vi "main(Test DQMH modules).vi"() -> ()   [LabVIEW 2018, in "Application.lvlib"] (continued)
              n429 = property class="ColBox"(reference=w1006, "Value"=u32 10000536 ("DRV 1")) -> ()  [unwired: 1 in, 2 out]
            }
            n430 = Build Array("Test Channel 2", "MEAS.AllRelaysOFF") -> (w1001:string[])
            n431 = for {
              tunnel: [w1010] -> w1002 mode=indexing
              tunnel: w1001 -> [w1009] mode=indexing
              tunnel: w1000 -> [w1008]
              n432 = call "App enquece.vi"("command"=w1009, "queue in"=w1008) -> ("error out"=w1010:errorcluster)  [unwired: 8 in, 1 out]
            }
            n433 = Merge Errors(w1004, w1002) -> (w1003:errorcluster)
          }
          event "Test Channel 3": Value Change {
            n434 = event-data() -> ()  [unwired: 1 in, 1 out]
            n435 = Array Subset(array=w1015, index=12, length=6) -> (w1016:refnum<vi>[])
            n436 = for {
              tunnel: w1016 -> [w1027] mode=indexing
              n437 = property class="ColBox"(reference=w1027, "Value"=u32 10000536 ("DRV 1")) -> ()  [unwired: 1 in, 2 out]
            }
            n438 = Build Array("Test Channel 3", "MEAS.AllRelaysOFF") -> (w1022:string[])
            n439 = for {
              tunnel: [w1031] -> w1023 mode=indexing
              tunnel: w1022 -> [w1030] mode=indexing
              tunnel: w1021 -> [w1029]
              n440 = call "App enquece.vi"("command"=w1030, "queue in"=w1029) -> ("error out"=w1031:errorcluster)  [unwired: 8 in, 1 out]
            }
            n441 = Merge Errors(w1025, w1023) -> (w1024:errorcluster)
          }
          event "Test Channel 4": Value Change {
            n442 = event-data() -> ()  [unwired: 1 in, 1 out]
            n443 = Array Subset(array=w1036, index=18, length=6) -> (w1037:refnum<vi>[])
            n444 = for {
              tunnel: w1037 -> [w1048] mode=indexing
              n445 = property class="ColBox"(reference=w1048, "Value"=u32 10000536 ("DRV 1")) -> ()  [unwired: 1 in, 2 out]
            }
            n446 = Build Array("Test Channel 4", "MEAS.AllRelaysOFF") -> (w1043:string[])
            n447 = for {
              tunnel: [w1052] -> w1044 mode=indexing
              tunnel: w1043 -> [w1051] mode=indexing
              tunnel: w1042 -> [w1050]
              n448 = call "App enquece.vi"("command"=w1051, "queue in"=w1050) -> ("error out"=w1052:errorcluster)  [unwired: 8 in, 1 out]
            }
            n449 = Merge Errors(w1046, w1044) -> (w1045:errorcluster)
          }
          event "Test Channel 5": Value Change {
            n450 = event-data() -> ()  [unwired: 1 in, 1 out]
            n451 = Array Subset(array=w1057, index=24, length=6) -> (w1058:refnum<vi>[])
            n452 = for {
              tunnel: w1058 -> [w1069] mode=indexing
              n453 = property class="ColBox"(reference=w1069, "Value"=u32 10000536 ("DRV 1")) -> ()  [unwired: 1 in, 2 out]
            }
            n454 = Build Array("Test Channel 5", "MEAS.AllRelaysOFF") -> (w1064:string[])
            n455 = for {
              tunnel: [w1073] -> w1065 mode=indexing
              tunnel: w1064 -> [w1072] mode=indexing
              tunnel: w1063 -> [w1071]
              n456 = call "App enquece.vi"("command"=w1072, "queue in"=w1071) -> ("error out"=w1073:errorcluster)  [unwired: 8 in, 1 out]
            }
            n457 = Merge Errors(w1067, w1065) -> (w1066:errorcluster)
          }
          event "Test Channel 6": Value Change {
            n458 = event-data() -> ()  [unwired: 1 in, 1 out]
            n459 = Array Subset(array=w1078, index=30, length=6) -> (w1079:refnum<vi>[])
            n460 = for {
              tunnel: w1079 -> [w1090] mode=indexing
              n461 = property class="ColBox"(reference=w1090, "Value"=u32 10000536 ("DRV 1")) -> ()  [unwired: 1 in, 2 out]
            }
            n462 = Build Array("Test Channel 6", "MEAS.AllRelaysOFF") -> (w1085:string[])
            n463 = for {
              tunnel: [w1094] -> w1086 mode=indexing
              tunnel: w1085 -> [w1093] mode=indexing
              tunnel: w1084 -> [w1092]
              n464 = call "App enquece.vi"("command"=w1093, "queue in"=w1092) -> ("error out"=w1094:errorcluster)  [unwired: 8 in, 1 out]
            }
            n465 = Merge Errors(w1088, w1086) -> (w1087:errorcluster)
          }
          event "Test Channel 7": Value Change {
            n466 = event-data() -> ()  [unwired: 1 in, 1 out]
            n467 = Array Subset(array=w1099, index=36, length=6) -> (w1100:refnum<vi>[])
            n468 = for {
              tunnel: w1100 -> [w1111] mode=indexing
              n469 = property class="ColBox"(reference=w1111, "Value"=u32 10000536 ("DRV 1")) -> ()  [unwired: 1 in, 2 out]
            }
            n470 = Build Array("Test Channel 7", "MEAS.AllRelaysOFF") -> (w1107:string[])
            n471 = for {
              tunnel: [w1115] -> w1103 mode=indexing
              tunnel: w1107 -> [w1114] mode=indexing
              tunnel: w1106 -> [w1113]
              n472 = call "App enquece.vi"("command"=w1114, "queue in"=w1113) -> ("error out"=w1115:errorcluster)  [unwired: 8 in, 1 out]
            }
            n473 = Merge Errors(w1109, w1103) -> (w1108:errorcluster)
          }
          event "Test Channel 8": Value Change {
            n474 = event-data() -> ()  [unwired: 1 in, 1 out]
            n475 = Array Subset(array=w1120, index=42, length=6) -> (w1121:refnum<vi>[])
            n476 = for {
              tunnel: w1121 -> [w1132] mode=indexing
              n477 = property class="ColBox"(reference=w1132, "Value"=u32 10000536 ("DRV 1")) -> ()  [unwired: 1 in, 2 out]
            }
            n478 = Build Array("Test Channel 8", "MEAS.AllRelaysOFF") -> (w1127:string[])
            n479 = for {
              tunnel: [w1136] -> w1128 mode=indexing
              tunnel: w1127 -> [w1135] mode=indexing
              tunnel: w1126 -> [w1134]
              n480 = call "App enquece.vi"("command"=w1135, "queue in"=w1134) -> ("error out"=w1136:errorcluster)  [unwired: 8 in, 1 out]
            }
            n481 = Merge Errors(w1130, w1128) -> (w1129:errorcluster)
          }
          event "Test Channel 9": Value Change {
            n482 = event-data() -> ()  [unwired: 1 in, 1 out]
            n483 = Array Subset(array=w1141, index=48, length=6) -> (w1142:refnum<vi>[])
            n484 = for {
              tunnel: w1142 -> [w1153] mode=indexing
              n485 = property class="ColBox"(reference=w1153, "Value"=u32 10000536 ("DRV 1")) -> ()  [unwired: 1 in, 2 out]
            }
            n486 = Build Array("Test Channel 9", "MEAS.AllRelaysOFF") -> (w1148:string[])
            n487 = for {
              tunnel: [w1157] -> w1149 mode=indexing
              tunnel: w1148 -> [w1156] mode=indexing
              tunnel: w1147 -> [w1155]
              n488 = call "App enquece.vi"("command"=w1156, "queue in"=w1155) -> ("error out"=w1157:errorcluster)  [unwired: 8 in, 1 out]
            }
            n489 = Merge Errors(w1151, w1149) -> (w1150:errorcluster)
          }
          event "Test Channel 10": Value Change {
            n490 = event-data() -> ()  [unwired: 1 in, 1 out]
            n491 = Array Subset(array=w1162, index=54, length=6) -> (w1163:refnum<vi>[])
            n492 = for {
              tunnel: w1163 -> [w1174] mode=indexing
              n493 = property class="ColBox"(reference=w1174, "Value"=u32 10000536 ("DRV 1")) -> ()  [unwired: 1 in, 2 out]
            }
            n494 = Build Array("Test Channel 10", "MEAS.AllRelaysOFF") -> (w1169:string[])
            n495 = for {
              tunnel: [w1178] -> w1170 mode=indexing
              tunnel: w1169 -> [w1177] mode=indexing
              tunnel: w1168 -> [w1176]
              n496 = call "App enquece.vi"("command"=w1177, "queue in"=w1176) -> ("error out"=w1178:errorcluster)  [unwired: 8 in, 1 out]
            }
            n497 = Merge Errors(w1172, w1170) -> (w1171:errorcluster)
          }
          event User Event {
            n498 = event-data() -> ("Init?"=w1182:bool)  [unwired: 1 in]
            "DC Measure Module" <- w1182
            "Inst. 1" <- w1182
            n499 = disable-structure shown="LOGGING==TRUE" {
              disable-tunnel: w1185 -> [w1192 _]
              frame condition #0 (active) {
                n500 = Empty String/Path?(string/path=w1192) -> (empty?=w1199:bool)
                n501 = Select(t="Quece timeout", s=w1199, f=w1192) -> (s? t:f=w1197:string)
                n502 = Format Into String(format string=":%s", initial string=w1197, "DMM  Did  it") -> (resulting string=w1194:string)  [unwired: 1 in, 1 out]
                n503 = call "string log (SubVI).vi"("Enum"=enum16{"Init", "Log", "Read"}."Log", "state Name"=w1194) -> ()  [unwired: 8 in, 2 out]
              }
              frame condition #1 {
              }
            }
            n504 = call "FGV Init phase.vi"("Boolean"=w1182) -> ("Init Completed?"=w1181:bool)  [unwired: 9 in, 1 out]
            n505 = case shown="True" w1181 {
              tunnel: w1180 -> [_ w1191]
              frame False {
              }
              frame True {
                n506 = call "App enquece.vi"("command"="INIT.Read DRV code", "queue in"=w1191) -> ()  [unwired: 8 in, 2 out]
              }
            }
            n507 = disable-structure shown="DEBUGGING==TRUE" {
              disable-tunnel: [w1200 w1202] -> w1187
              disable-tunnel: w1186 -> [w1200 w1203]
              frame condition #0 (active) {
              }
              frame condition #1 {
                n508 = call "Show Panel.vi"() -> ("error out"=w1201:errorcluster)  [unwired: 11 in]
                n509 = Merge Errors(w1203, w1201) -> (w1202:errorcluster)
              }
            }
          }
          event User Event {
            n510 = event-data() -> ("Init?"=w1207:bool)  [unwired: 1 in]
            "AC switches Module" <- w1207
            "Inst. 2" <- w1207
            n511 = disable-structure shown="LOGGING==TRUE" {
              disable-tunnel: w1212 -> [w1221 _]
              frame condition #0 (active) {
                n512 = Empty String/Path?(string/path=w1221) -> (empty?=w1228:bool)
                n513 = Select(t="Quece timeout", s=w1228, f=w1221) -> (s? t:f=w1226:string)
                n514 = Format Into String(format string=":%s", initial string=w1226, "MB01  Did  it") -> (resulting string=w1223:string)  [unwired: 1 in, 1 out]
                n515 = call "string log (SubVI).vi"("Enum"=enum16{"Init", "Log", "Read"}."Log", "state Name"=w1223) -> ()  [unwired: 8 in, 2 out]
              }
              frame condition #1 {
              }
            }
            n516 = call "FGV Init phase.vi"("Boolean"=w1207) -> ("Init Completed?"=w1206:bool)  [unwired: 9 in, 1 out]
            n517 = disable-structure shown="DEBUGGING==TRUE" {
              disable-tunnel: [w1217 w1220] -> w1211
              disable-tunnel: w1210 -> [w1217 w1219]
              frame condition #0 (active) {
              }
              frame condition #1 {
                n518 = call "Show Panel.vi"() -> ("error out"=w1218:errorcluster)  [unwired: 11 in]
                n519 = Merge Errors(w1219, w1218) -> (w1220:errorcluster)
              }
            }
            n520 = case shown="True" w1206 {
              tunnel: w1205 -> [_ w1215]
              frame False {
              }
              frame True {
                n521 = call "App enquece.vi"("command"="INIT.Read DRV code", "queue in"=w1215) -> ()  [unwired: 8 in, 2 out]
              }
            }
          }
          event User Event {
            n522 = event-data() -> ("Init?"=w1232:bool)  [unwired: 1 in]
            "DC Switches Module" <- w1232
            "Inst. 3" <- w1232
            n523 = disable-structure shown="LOGGING==TRUE" {
              disable-tunnel: w1235 -> [w1242 _]
              frame condition #0 (active) {
                n524 = Empty String/Path?(string/path=w1242) -> (empty?=w1249:bool)
                n525 = Select(t="Quece timeout", s=w1249, f=w1242) -> (s? t:f=w1247:string)
                n526 = Format Into String(format string=":%s", initial string=w1247, "M054  Did  it") -> (resulting string=w1244:string)  [unwired: 1 in, 1 out]
                n527 = call "string log (SubVI).vi"("Enum"=enum16{"Init", "Log", "Read"}."Log", "state Name"=w1244) -> ()  [unwired: 8 in, 2 out]
              }
              frame condition #1 {
              }
            }
            n528 = call "FGV Init phase.vi"("Boolean"=w1232) -> ("Init Completed?"=w1231:bool)  [unwired: 9 in, 1 out]
            n529 = case shown="True" w1231 {
              tunnel: w1230 -> [_ w1240]
              frame False {
              }
              frame True {
                n530 = call "App enquece.vi"("command"="INIT.Read DRV code", "queue in"=w1240) -> ()  [unwired: 8 in, 2 out]
              }
            }
            n531 = disable-structure shown="DEBUGGING==TRUE" {
              disable-tunnel: w1237 -> [w1250 w1252 w1255]
              disable-tunnel: [w1251 w1252 w1253] -> w1236
              frame condition #0 (active) {
                n532 = Merge Errors(w1250) -> (w1251:errorcluster)
              }
              frame condition #1 {
              }
              frame condition #2 {
                n533 = call "Show Panel.vi"() -> ("error out"=w1254:errorcluster)  [unwired: 11 in]
                n534 = Merge Errors(w1255, w1254) -> (w1253:errorcluster)
              }
            }
          }
        }
      }
      frame "Apps.AutoMode" {
        # "Check Jig trigger every 100ms"
        n535 = disable-structure shown="Enabled" {
          frame Disabled {
            n536 = local write "Auto/Man"(TRUE) -> ()
          }
          frame Enabled {
          }
        }
      }
      frame "Apps.WaitingForTrigger" {
        n537 = call "App enquece.vi"("command"="MEAS.Read TRIGGER", "queue in"=w1270) -> ("error out"=w1268:errorcluster)  [unwired: 8 in, 1 out]
        n538 = Merge Errors(w1266, w1268) -> (w1267:errorcluster)
      }
      frame "Apps.UpdateStatus" {
        n539 = disable-structure shown="LOGGING==TRUE" {
          disable-tunnel: w1278 -> [w1291 _]
          frame condition #0 (active) {
            n540 = Empty String/Path?(string/path=w1291) -> (empty?=w1294:bool)
            n541 = Select(t="Quece timeout", s=w1294, f=w1291) -> (s? t:f=w1290:string)
            n542 = call "string log (SubVI).vi"("Enum"=enum16{"Init", "Log", "Read"}."Log", "state Name"=w1290) -> ()  [unwired: 8 in, 2 out]
          }
          frame condition #1 {
          }
        }
        n543 = call "App enquece.vi"("command"="Apps.WaitForEvent", "queue in"=w1286) -> ("error out"=w1283:errorcluster)  [unwired: 8 in, 1 out]
        n544 = Merge Errors(w1279, w1283) -> (w1280:errorcluster)
      }
      frame "Apps.UI Update" {
        # "Update UI  6LED (channel)"
        n545 = disable-structure shown="LOGGING==TRUE" {
          disable-tunnel: w1298 -> [w1418 _]
          frame condition #0 (active) {
            n546 = Empty String/Path?(string/path=w1418) -> (empty?=w1421:bool)
            n547 = Select(t="Quece timeout", s=w1421, f=w1418) -> (s? t:f=w1417:string)
            n548 = call "string log (SubVI).vi"("Enum"=enum16{"Init", "Log", "Read"}."Log", "state Name"=w1417) -> ()  [unwired: 8 in, 2 out]
          }
          frame condition #1 {
          }
        }
        n549 = Variant To Data(type="", Variant=w1296) -> (data=w1295:string)  [unwired: 1 in, 1 out]
        n550 = case shown="\"A\"" w1295 {
          tunnel: [w1319 w1327 w1345 w1363 w1381 w1399] -> w1304
          tunnel: w1302 -> [w1317 w1328 w1346 w1364 w1382 w1400]
          tunnel: w1301 -> [w1314 w1329 w1347 w1365 w1383 w1401]
          frame "", Default {
            w1311 = 6 ("length")
            n551 = call "FGV Driver Data.vi"("DUT channel (1-11)"=w1314, "FGV enum(Read)"=FGV_DRV_data."Process" ("FGV DRV data enum")) -> ("60 DRV data"=w1312:T17[])  [unwired: 6 in, 3 out]
            n552 = Decrement(x=w1314) -> (x-1=w1315:i32)
            n553 = Multiply(x=w1315, y=w1311) -> (x*y=w1313:i32)
            n554 = Array Subset(array=w1312, index=w1313, length=w1311) -> (w1310:T17[])
            n555 = Array Subset(array=w1317, index=w1313, length=w1311) -> (w1316:refnum<vi>[])
            n556 = for {
              tunnel: w1316 -> [w1322] mode=indexing
              tunnel: w1310 -> [w1321] mode=indexing
              tunnel: [w1320] -> w1319 mode=indexing
              n557 = Unbundle By Name(w1321) -> ("DRV Fail/Pass (T)"=w1325:bool)
              n558 = Select(t=u32 16711686 ("DRV 1"), s=w1325, f=u32 65309 ("DRV 1")) -> (s? t:f=w1326:u32)
              n559 = property class="ColBox"(reference=w1322, "Value"=w1326) -> (error out=w1320:errorcluster)  [unwired: 1 in, 1 out]
            }
          }
          frame "A" {
            w1330 = 1
            n560 = call "FGV Driver Data.vi"("DUT channel (1-11)"=w1329, "FGV enum(Read)"=FGV_DRV_data."Process" ("FGV DRV data enum")) -> ("60 DRV data"=w1333:T17[])  [unwired: 6 in, 3 out]
            n561 = Decrement(x=w1329) -> (x-1=w1335:i32)
            n562 = Multiply(x=w1335, y=6 ("length")) -> (x*y=w1334:i32)
            n563 = Array Subset(array=w1333, index=w1334, length=w1330) -> (w1331:T17[])
            n564 = Array Subset(array=w1328, index=w1334, length=w1330) -> (w1336:refnum<vi>[])
            n565 = for {
              tunnel: w1336 -> [w1340] mode=indexing
              tunnel: w1331 -> [w1339] mode=indexing
              tunnel: [w1338] -> w1327 mode=indexing
              n566 = Unbundle By Name(w1339) -> ("DRV Fail/Pass (T)"=w1343:bool)
              n567 = Select(t=u32 16711686 ("DRV 1"), s=w1343, f=u32 65309 ("DRV 1")) -> (s? t:f=w1344:u32)
              n568 = property class="ColBox"(reference=w1340, "Value"=w1344) -> (error out=w1338:errorcluster)  [unwired: 1 in, 1 out]
            }
          }
          frame "B" {
            w1348 = 2
            n569 = call "FGV Driver Data.vi"("DUT channel (1-11)"=w1347, "FGV enum(Read)"=FGV_DRV_data."Process" ("FGV DRV data enum")) -> ("60 DRV data"=w1351:T17[])  [unwired: 6 in, 3 out]
            n570 = Decrement(x=w1347) -> (x-1=w1353:i32)
            n571 = Multiply(x=w1353, y=6 ("length")) -> (x*y=w1352:i32)
            n572 = Array Subset(array=w1351, index=w1352, length=w1348) -> (w1349:T17[])
            n573 = Array Subset(array=w1346, index=w1352, length=w1348) -> (w1354:refnum<vi>[])
            n574 = for {
              tunnel: w1354 -> [w1358] mode=indexing
              tunnel: w1349 -> [w1357] mode=indexing
              tunnel: [w1356] -> w1345 mode=indexing
              n575 = Unbundle By Name(w1357) -> ("DRV Fail/Pass (T)"=w1361:bool)
              n576 = Select(t=u32 16711686 ("DRV 1"), s=w1361, f=u32 65309 ("DRV 1")) -> (s? t:f=w1362:u32)
              n577 = property class="ColBox"(reference=w1358, "Value"=w1362) -> (error out=w1356:errorcluster)  [unwired: 1 in, 1 out]
            }
          }
          frame "C" {
            w1366 = 3
            n578 = call "FGV Driver Data.vi"("DUT channel (1-11)"=w1365, "FGV enum(Read)"=FGV_DRV_data."Process" ("FGV DRV data enum")) -> ("60 DRV data"=w1369:T17[])  [unwired: 6 in, 3 out]
            n579 = Decrement(x=w1365) -> (x-1=w1371:i32)
            n580 = Multiply(x=w1371, y=6 ("length")) -> (x*y=w1370:i32)
            n581 = Array Subset(array=w1369, index=w1370, length=w1366) -> (w1367:T17[])
            n582 = Array Subset(array=w1364, index=w1370, length=w1366) -> (w1372:refnum<vi>[])
            n583 = for {
              tunnel: w1372 -> [w1376] mode=indexing
              tunnel: w1367 -> [w1375] mode=indexing
              tunnel: [w1374] -> w1363 mode=indexing
              n584 = Unbundle By Name(w1375) -> ("DRV Fail/Pass (T)"=w1379:bool)
              n585 = Select(t=u32 16711686 ("DRV 1"), s=w1379, f=u32 65309 ("DRV 1")) -> (s? t:f=w1380:u32)
              n586 = property class="ColBox"(reference=w1376, "Value"=w1380) -> (error out=w1374:errorcluster)  [unwired: 1 in, 1 out]
            }
          }
          frame "D" {
            w1384 = 4
            n587 = call "FGV Driver Data.vi"("DUT channel (1-11)"=w1383, "FGV enum(Read)"=FGV_DRV_data."Process" ("FGV DRV data enum")) -> ("60 DRV data"=w1387:T17[])  [unwired: 6 in, 3 out]
            n588 = Decrement(x=w1383) -> (x-1=w1389:i32)
            n589 = Multiply(x=w1389, y=6 ("length")) -> (x*y=w1388:i32)
            n590 = Array Subset(array=w1387, index=w1388, length=w1384) -> (w1385:T17[])
            n591 = Array Subset(array=w1382, index=w1388, length=w1384) -> (w1390:refnum<vi>[])
            n592 = for {
              tunnel: w1390 -> [w1394] mode=indexing
              tunnel: w1385 -> [w1393] mode=indexing
              tunnel: [w1392] -> w1381 mode=indexing
              n593 = Unbundle By Name(w1393) -> ("DRV Fail/Pass (T)"=w1397:bool)
              n594 = Select(t=u32 16711686 ("DRV 1"), s=w1397, f=u32 65309 ("DRV 1")) -> (s? t:f=w1398:u32)
              n595 = property class="ColBox"(reference=w1394, "Value"=w1398) -> (error out=w1392:errorcluster)  [unwired: 1 in, 1 out]
            }
          }
          frame "E" {
            w1402 = 5
            n596 = call "FGV Driver Data.vi"("DUT channel (1-11)"=w1401, "FGV enum(Read)"=FGV_DRV_data."Process" ("FGV DRV data enum")) -> ("60 DRV data"=w1405:T17[])  [unwired: 6 in, 3 out]
            n597 = Decrement(x=w1401) -> (x-1=w1407:i32)
            n598 = Multiply(x=w1407, y=6 ("length")) -> (x*y=w1406:i32)
            n599 = Array Subset(array=w1405, index=w1406, length=w1402) -> (w1403:T17[])
            n600 = Array Subset(array=w1400, index=w1406, length=w1402) -> (w1408:refnum<vi>[])
            n601 = for {
              tunnel: w1408 -> [w1412] mode=indexing
              tunnel: w1403 -> [w1411] mode=indexing
              tunnel: [w1410] -> w1399 mode=indexing
              n602 = Unbundle By Name(w1411) -> ("DRV Fail/Pass (T)"=w1415:bool)
              n603 = Select(t=u32 16711686 ("DRV 1"), s=w1415, f=u32 65309 ("DRV 1")) -> (s? t:f=w1416:u32)
              n604 = property class="ColBox"(reference=w1412, "Value"=w1416) -> (error out=w1410:errorcluster)  [unwired: 1 in, 1 out]
            }
          }
        }
        n605 = Merge Errors(w1305, w1304) -> (w1306:errorcluster)
      }
      frame "Apps.UI Update 1" {
        # "For Update UI 1 LED"
        n606 = disable-structure shown="LOGGING==TRUE" {
          disable-tunnel: w1436 -> [w1444 _]
          frame condition #0 (active) {
            n607 = Empty String/Path?(string/path=w1444) -> (empty?=w1447:bool)
            n608 = Select(t="Quece timeout", s=w1447, f=w1444) -> (s? t:f=w1443:string)
            n609 = call "string log (SubVI).vi"("Enum"=enum16{"Init", "Log", "Read"}."Log", "state Name"=w1443) -> ()  [unwired: 8 in, 2 out]
          }
          frame condition #1 {
          }
        }
        n610 = call "FGV Driver Data.vi"("DUT channel (1-11)"=w1434, "FGV enum(Read)"=FGV_DRV_data."Process" ("FGV DRV data enum")) -> ("60 DRV data"=w1427:T17[])  [unwired: 6 in, 3 out]
        n611 = Decrement(x=w1422) -> (x-1=w1423:i32)
        n612 = Index Array(array=w1428, index=w1423) -> (element=w1425:refnum<vi>)
        n613 = Index Array(array=w1427, index=w1423) -> (element=w1426:T17)
        n614 = Unbundle By Name(w1426) -> ("DRV Fail/Pass (T)"=w1424:bool)
        n615 = Select(t=u32 16711686 ("DRV 1"), s=w1424, f=u32 65309 ("DRV 1")) -> (s? t:f=w1431:u32)
        n616 = property class="ColBox"(reference=w1425, "Value"=w1431) -> (error out=w1437:errorcluster)  [unwired: 1 in, 1 out]
        n617 = Merge Errors(w1438, w1437) -> (w1439:errorcluster)
      }
      frame "Apps.UI Update 2" {
        # "For Updat PCB OK/NG (1 LED)"
        n618 = local read "Auto/Man"() -> (w1455:bool)
        n619 = disable-structure shown="LOGGING==TRUE" {
          disable-tunnel: w1468 -> [w1510 _]
          frame condition #0 (active) {
            n620 = Empty String/Path?(string/path=w1510) -> (empty?=w1513:bool)
            n621 = Select(t="Quece timeout", s=w1513, f=w1510) -> (s? t:f=w1509:string)
            n622 = call "string log (SubVI).vi"("Enum"=enum16{"Init", "Log", "Read"}."Log", "state Name"=w1509) -> ()  [unwired: 8 in, 2 out]
          }
          frame condition #1 {
          }
        }
        n623 = case shown="True" w1455 {
          tunnel: w1460 -> [_ w1502]
          tunnel: [_ w1501] -> w1459
          frame False {
          }
          frame True {
            n624 = call "App enquece.vi"("command"="Apps.AutoMode", "queue in"=w1502) -> ("error out"=w1501:errorcluster)  [unwired: 8 in, 1 out]
          }
        }
        n625 = call "FGV Driver Data.vi"("error in (no error)"=w1459, "FGV enum(Read)"=FGV_DRV_data."Process" ("FGV DRV data enum")) -> ("error out"=w1467:errorcluster, "60 DRV data"=w1464:T17[])  [unwired: 6 in, 2 out]
        n626 = call "FGV DUT steps.vi"("Enum"=enum16{"write", "read"}."read") -> ("Steps OUT"=w1452:string[])  [unwired: 10 in]
        n627 = Index Array(array=w1452, index=1) -> (element=w1453:string)
        n628 = Decimal String To Number(string=w1453) -> (number=w1450:i32)  [unwired: 2 in, 1 out]
        n629 = call "find Index and length.vi"("number of DRV"=w1450) -> ("length"=w1448:i32, "index"=w1449:i32)  [unwired: 8 in, 1 out]
        n630 = disable-structure shown="Enabled" {
          disable-tunnel: w1464 -> [w1484 w1499]
          disable-tunnel: [w1482 w1498] -> w1457
          disable-tunnel: w1449 -> [_ w1497]
          disable-tunnel: w1448 -> [_ w1496]
          frame Disabled {
            n631 = local read "Enum"() -> (w1483:T1)
            n632 = case shown="\"00037845(M26)\"" w1483 {
              tunnel: w1484 -> [w1487 w1489 w1491 w1495]
              tunnel: [w1486 w1488 w1491 w1494] -> w1482
              frame "Fixxed", Default {
                n633 = Array Subset(array=w1487, length=41) -> (w1486:T17[])  [unwired: 1 in]
              }
              frame "Pinpoint_JIG" {
                n634 = Array Subset(array=w1489, index=42) -> (w1488:T17[])  [unwired: 1 in]
              }
              frame "All DRV" {
              }
              frame "00037845(M26)" {
                n635 = Array Subset(array=w1495, index=42, length=14) -> (w1494:T17[])
              }
            }
          }
          frame Enabled {
            n636 = Array Subset(array=w1499, index=w1497, length=w1496) -> (w1498:T17[])
          }
        }
        n637 = for {
          tunnel: w1457 -> [w1515] mode=indexing
          tunnel: [w1514] -> w1474 mode=indexing
          n638 = Unbundle By Name(w1515) -> ("DRV Fail/Pass (T)"=w1514:bool)
        }
        n639 = Or Array Elements(Boolean array=w1474) -> (logical OR=w1472:bool)
        n640 = control-ref of="DRV 61"() -> (w1473:refnum<vi>)
        n641 = Select(t=u32 16711680 ("DRV 1"), s=w1472, f=u32 6618880 ("DRV 1")) -> (s? t:f=w1469:u32)
        n642 = property class="ColBox"(reference=w1473, error in=w1467, "Value"=w1469) -> (error out=w1466:errorcluster)  [unwired: 1 out]
        n643 = case shown="False" "Log report" {
          tunnel: w1457 -> [_ w1504]
          tunnel: w1456 -> [_ w1505]
          frame False {
          }
          frame True {
            # "Log trigger"
            n644 = To Variant(anything=w1504) -> (Variant=w1503:variant)
            n645 = Enqueue Element(queue=w1505, element=w1503) -> ()  [unwired: 2 in, 3 out]
          }
        }
        n646 = Merge Errors(w1481, w1466) -> (w1461:errorcluster)
        n647 = disable-structure shown="NO_HARDWARE==TRUE" {
          disable-tunnel: [w1506 w1508] -> w1462
          disable-tunnel: w1461 -> [w1506 w1508]
          frame condition #0 (active) {
            n648 = Wait (ms)(milliseconds to wait=u32 2000) -> ()  [unwired: 1 out]
          }
          frame condition #1 {
          }
        }
      }
      frame "Apps.UI Update SC" {
        w1525 = "All Shorted Circuits"
        n649 = disable-structure shown="LOGGING==TRUE" {
          disable-tunnel: w1531 -> [w1576 _]
          frame condition #0 (active) {
            n650 = Empty String/Path?(string/path=w1576) -> (empty?=w1579:bool)
            n651 = Select(t="Quece timeout", s=w1579, f=w1576) -> (s? t:f=w1575:string)
            n652 = call "string log (SubVI).vi"("Enum"=enum16{"Init", "Log", "Read"}."Log", "state Name"=w1575) -> ()  [unwired: 8 in, 2 out]
          }
          frame condition #1 {
          }
        }
        n653 = call "FGV DUT steps.vi"("Enum"=enum16{"write", "read"}."read") -> ("Steps OUT"=w1517:string[])  [unwired: 10 in]
        n654 = Index Array(array=w1517, index=1) -> (element=w1519:string)
        n655 = call "FGV Driver Data.vi"("FGV enum(Read)"=FGV_DRV_data."Read" ("FGV DRV data enum")) -> ("60 DRV data"=w1522:T17[])  [unwired: 7 in, 3 out]
        n656 = Decimal String To Number(string=w1519) -> (number=w1518:i32)  [unwired: 2 in, 1 out]
        n657 = disable-structure shown="Enabled" {
          disable-tunnel: w1524 -> [w1544 w1568]
          disable-tunnel: [w1543 w1567] -> w1523
          disable-tunnel: w1522 -> [w1542 w1566]
          disable-tunnel: [w1541 w1563] -> w1521
          disable-tunnel: w1518 -> [_ w1569]
          frame Disabled {
            n658 = local read "Enum"() -> (w1540:T1)
            n659 = case shown="\"00037845(M26)\"" w1540 {
              tunnel: w1544 -> [w1549 w1554 w1556 w1561]
              tunnel: [w1548 w1550 w1556 w1559] -> w1543
              tunnel: w1542 -> [w1547 w1553 w1555 w1560]
              tunnel: [w1545 w1552 w1555 w1558] -> w1541
              frame "Fixxed", Default {
                w1546 = 42 ("length")
                n660 = Array Subset(array=w1547, length=w1546) -> (w1545:T17[])  [unwired: 1 in]
                n661 = Array Subset(array=w1549, length=w1546) -> (w1548:refnum<vi>[])  [unwired: 1 in]
              }
              frame "Pinpoint_JIG" {
                w1551 = 42 ("length")
                n662 = Array Subset(array=w1554, index=w1551) -> (w1550:refnum<vi>[])  [unwired: 1 in]
                n663 = Array Subset(array=w1553, index=w1551) -> (w1552:T17[])  [unwired: 1 in]
              }
              frame "All DRV" {
              }
              frame "00037845(M26)" {
                w1557 = 14 ("length")
                w1562 = 42 ("length")
                n664 = Array Subset(array=w1561, index=w1562, length=w1557) -> (w1559:refnum<vi>[])
                n665 = Array Subset(array=w1560, index=w1562, length=w1557) -> (w1558:T17[])
              }
            }
          }
          frame Enabled {
            n666 = call "find Index and length.vi"("number of DRV"=w1569) -> ("length"=w1564:i32, "index"=w1565:i32)  [unwired: 8 in, 1 out]
            n667 = Array Subset(array=w1568, index=w1565, length=w1564) -> (w1567:refnum<vi>[])
            n668 = Array Subset(array=w1566, index=w1565, length=w1564) -> (w1563:T17[])
          }
        }
        n669 = for {
          tunnel: w1521 -> [w1586] mode=indexing
          tunnel: w1523 -> [w1581] mode=indexing
          tunnel: [w1580] -> w1529 mode=indexing
          n670 = Unbundle By Name(w1586) -> ("Shorted Circuit"=w1582:bool)
          n671 = Select(t=u32 16711680 ("DRV 1"), s=w1582, f=u32 6618880 ("DRV 1")) -> (s? t:f=w1585:u32)
          n672 = property class="ColBox"(reference=w1581, "Value"=w1585) -> (error out=w1580:errorcluster)  [unwired: 1 in, 1 out]
        }
        n673 = Merge Errors(w1529) -> (w1528:errorcluster)
        n674 = flat-sequence {
          tunnel: w1528 -> [w1571]
          tunnel: [w1571] -> w1527
          tunnel: w1527 -> [w1573]
          tunnel: [w1574] -> w1526
          tunnel: w1524 -> [w1572]
          frame #0 {
            n675 = Wait (ms)(milliseconds to wait=u32 1500) -> ()  [unwired: 1 out]
          }
          frame #1 {
            n676 = call "reset DRV UI (SubVI).vi"("error in (no error)"=w1573, "Ref  in"=w1572) -> ("error out"=w1574:errorcluster)  [unwired: 8 in, 1 out]
          }
        }
        n677 = Merge Errors(w1539, w1526) -> (w1530:errorcluster)
        n678 = local write "Progress"(w1525) -> ()
      }
      frame "Timer Start" {
        n679 = flat-sequence {
          tunnel: [u32 0 ("time elased(ms)")] -> w1587
          frame #0 {
            n680 = call "FGV milisec (subVI).vi"() -> ()  [unwired: 11 in, 1 out]
          }
        }
        n681 = local write "time elased(ms)"(w1587) -> ()
      }
      frame "Timer Stop" {
        n682 = flat-sequence {
          tunnel: [w1608] -> w1597
          tunnel: w1598 -> [w1608]
          tunnel: [w1607] -> w1599
          frame #0 {
            n683 = call "FGV milisec (subVI).vi"() -> ("Elased Time (ms)"=w1607:u32)  [unwired: 11 in]
          }
        }
        "time elased(ms)" <- w1599
      }
      frame "WaitFor" {
        n684 = Variant To Data(type=u32 0, Variant=w1609) -> ()  [unwired: 1 in, 2 out]
        n685 = Wait (ms)(milliseconds to wait="milliseconds to wait") -> ()  [unwired: 1 out]
      }
      frame "Apps.Exit" {
        w1624 = TRUE
        n686 = disable-structure shown="LOGGING==TRUE" {
          disable-tunnel: w1621 -> [w1639 _]
          frame condition #0 (active) {
            n687 = Empty String/Path?(string/path=w1639) -> (empty?=w1642:bool)
            n688 = Select(t="Quece timeout", s=w1642, f=w1639) -> (s? t:f=w1638:string)
            n689 = call "string log (SubVI).vi"("Enum"=enum16{"Init", "Log", "Read"}."Log", "state Name"=w1638) -> ()  [unwired: 8 in, 2 out]
          }
          frame condition #1 {
          }
        }
        n690 = call "Application Name--constant.vi"() -> ("Application Name"=w1625:string)  [unwired: 11 in]
        n691 = call "Stop Module.vi"("Wait for Module to stop? (F)"=w1624, "Origin"=w1625, "Module ID"=-1) -> ("error out"=w1627:errorcluster)  [unwired: 8 in]
        n692 = call "Stop Module.vi"("Wait for Module to Stop? (F)"=w1624, "Origin"=w1625) -> ("error out"=w1633:errorcluster)  [unwired: 9 in]
        n693 = call "Stop Module.vi"("Wait for Module to Stop? (F)"=w1624, "Origin"=w1625) -> ("error out"=w1632:errorcluster)  [unwired: 9 in]
        n694 = call "Stop Module.vi"("Wait for Module to Stop? (F)"=w1624, "Origin"=w1625) -> ("error out"=w1631:errorcluster)  [unwired: 9 in]
        n695 = Merge Errors(w1629, w1633, w1632, w1631, w1627) -> (w1630:errorcluster)
      }
      frame "Apps.Error Handler" {
        w1651 = TRUE  # Priority Enquece
        n696 = disable-structure shown="LOGGING==TRUE" {
          disable-tunnel: w1644 -> [w1660 _]
          frame condition #0 (active) {
            n697 = Empty String/Path?(string/path=w1660) -> (empty?=w1663:bool)
            n698 = Select(t="Quece timeout", s=w1663, f=w1660) -> (s? t:f=w1659:string)
            n699 = call "string log (SubVI).vi"("Enum"=enum16{"Init", "Log", "Read"}."Log", "state Name"=w1659) -> ()  [unwired: 8 in, 2 out]
          }
          frame condition #1 {
          }
        }
        n700 = call <vilib>:"Simple Error Handler.vi"("error in (no error)"=w1658) -> ("error out"=w1653:errorcluster)  [unwired: 4 in, 4 out]
        n701 = flat-sequence {
          tunnel: w1653 -> [_]
          tunnel: [w1664] -> w1645
          frame #0 {
            n702 = xnode "Error Ring"() -> ("error out"=w1664:errorcluster)
          }
        }
        n703 = call "App enquece.vi"("Priority Enquece"=w1651, "command"="Apps.Exit", "queue in"=w1652) -> ("error out"=w1650:errorcluster)  [unwired: 7 in, 1 out]
        n704 = Merge Errors(w1645, w1650) -> (w1646:errorcluster)
      }
      frame "INIT.Init FGV" {
        n705 = call "FGV_HoldingRegs.vi"("FGV_enum"=FGV_enum."Init FGV") -> ("error out"=w1670:errorcluster)  [unwired: 8 in, 2 out]
        n706 = call "string log (SubVI).vi"("error in (no error)"=w1670, "Enum"=enum16{"Init", "Log", "Read"}."Init") -> ("error out"=w1671:errorcluster)  [unwired: 8 in, 1 out]
        n707 = call "FGV Driver Data.vi"("error in (no error)"=w1671, "FGV enum(Read)"=FGV_DRV_data."Init" ("FGV DRV data enum")) -> ("error out"=w1668:errorcluster)  [unwired: 6 in, 3 out]
        n708 = call "FGV Init phase.vi"("error in (no error)"=w1668, "FGV Enum"=enum16{"Init", "Check"}."Init") -> ("error out"=w1666:errorcluster)  [unwired: 8 in, 1 out]
        n709 = flat-sequence {
          tunnel: [w1684] -> w1667
          tunnel: w1666 -> [w1684]
          frame #0 {
            n710 = Initialize Array(FALSE, 6 ("dimension size"), 10 ("dimension size")) -> (w1688:bool[][])
            n711 = local write "EMIC connected"(bool[] [FALSE, FALSE, FALSE, FALSE, FALSE, FALSE] ("Array")) -> ()
            n712 = local write "Auto/Man"(FALSE) -> ()
            n713 = local write "Short DRV"(w1688) -> ()
          }
        }
        n714 = Merge Errors(w1683, w1667) -> (w1673:errorcluster)
      }
      frame "INIT.Read HW config" {
        n715 = disable-structure shown="LOGGING==TRUE" {
          disable-tunnel: w1703 -> [w1729 _]
          frame condition #0 (active) {
            n716 = Empty String/Path?(string/path=w1729) -> (empty?=w1732:bool)
            n717 = Select(t="Quece timeout", s=w1732, f=w1729) -> (s? t:f=w1728:string)
            n718 = call "string log (SubVI).vi"("Enum"=enum16{"Init", "Log", "Read"}."Log", "state Name"=w1728) -> ()  [unwired: 8 in, 2 out]
          }
          frame condition #1 {
          }
        }
        n719 = disable-structure shown="RUN_TIME_ENGINE==True" {
          disable-tunnel: ["Development" ("version") "v5.0 Released"] -> w1702
          frame condition #0 (active) {
          }
          frame condition #1 {
          }
        }
        "version" <- w1702
        n720 = call <vilib>:"Application Directory.vi"() -> ("Application Directory"=w1698:path)
        n721 = Build Path(base path=w1698, name or relative path="config") -> (appended path=w1697:path)
        n722 = call "HW Config.vi"("start path"=w1697) -> ("error out"=w1704:errorcluster, "HW config 2"=w1711:T9)  [unwired: 9 in]
        n723 = Bundle By Name(cluster=w1712, "HW config 2"=w1711) -> (w1710:cluster{"HW config 2":T9})
        n724 = invoke class="VI" method="FP.Open"(error in=w1704, "State"=T18."Minimized") -> (error out=w1693:errorcluster)  [unwired: 3 in, 4 out]
        n725 = call "Login.vi"("error in (no error)"=w1693) -> ("error out"=w1695:errorcluster, "Login Successed"=w1696:bool, "UserName"=w1692:string)  [unwired: 8 in]
        n726 = call "FGV _Operator Name.vi"("Enum"=enum16{"Write", "Read"}."Write", "Operator Name in"=w1692) -> ()  [unwired: 9 in, 1 out]
        n727 = case shown="False" w1696 {
          tunnel: w1700 -> [w1722 _]
          tunnel: w1695 -> [w1719 w1724]
          tunnel: [w1718 w1725] -> w1705
          frame False {
            n728 = call "string log (SubVI).vi"("Enum"=enum16{"Init", "Log", "Read"}."Init") -> ("error out"=w1716:errorcluster)  [unwired: 9 in, 1 out]
            n729 = call "App enquece.vi"("Priority Enquece"=TRUE, "error in (no error)"=w1719, "command"="Apps.Exit", "queue in"=w1722) -> ("error out"=w1718:errorcluster)  [unwired: 6 in, 1 out]
            n730 = call "inst.InitialiseFGV.vi"("error in (no error)"=w1716) -> ()  [unwired: 10 in, 1 out]
          }
          frame True {
            n731 = invoke class="VI" method="FP.Open"(error in=w1724, "State"=T18."Standard") -> (error out=w1725:errorcluster)  [unwired: 3 in, 4 out]
          }
        }
        n732 = Merge Errors(w1715, w1705) -> (w1706:errorcluster)
      }
      frame "INIT.Read DRV code" {
        w1763 = u8 2 items=["SLOW", "MID", "FAST"] ("Detector Rate")
        # "Convert from [mA] to [A]"
        n733 = disable-structure shown="LOGGING==TRUE" {
          disable-tunnel: w1771 -> [w1781 _]
          frame condition #0 (active) {
            n734 = Empty String/Path?(string/path=w1781) -> (empty?=w1784:bool)
            n735 = Select(t="Quece timeout", s=w1784, f=w1781) -> (s? t:f=w1780:string)
            n736 = call "string log (SubVI).vi"("Enum"=enum16{"Init", "Log", "Read"}."Log", "state Name"=w1780) -> ()  [unwired: 8 in, 2 out]
          }
          frame condition #1 {
          }
        }
        n737 = invoke class="VI" method="FP.Open"("State"=T18."Hidden") -> (error out=w1748:errorcluster)  [unwired: 4 in, 4 out]
        n738 = call "ReadDriverParameters.vi"("error in (no error)"=w1748) -> ("error out"=w1746:errorcluster, "DRV stand"=w1754:T2)  [unwired: 9 in]
        n739 = invoke class="VI" method="FP.Open"(error in=w1746, "State"=T18."Standard") -> (error out=w1750:errorcluster)  [unwired: 3 in, 4 out]
        n740 = Merge Errors(w1772, w1750) -> (w1773:errorcluster)
        n741 = call "FGV DRV stand.vi"("Enum"=enum16{"Write", "Read"}."Write", "DRV stand  in"=w1754) -> ("DRV stand out"=w1751:T2)  [unwired: 9 in]
        "DRV stand" <- w1751
        n742 = Unbundle By Name(w1751) -> ("SAP ID"=w1739:string, "Name"=w1740:string)
        "SAP ID" <- w1739
        "Name" <- w1740
        n743 = Unbundle By Name(w1754) -> ("DC characteristics.Voltage.Max"=w1745:dbl, "DC characteristics.Current.Max"=w1770:dbl)
        n744 = call "FGV SapID & Name.vi"("Enum"=enum16{"Read", "Write"}."Write", "Name"=w1740, "SAP ID"=w1739) -> ("SAP ID out"=w1736:string)  [unwired: 7 in, 1 out]
        n745 = Divide(x=w1770, y=1000.0) -> (x/y=w1742:dbl)
        n746 = call "FGV DUT steps.vi"("Enum"=enum16{"write", "read"}."write", "SapID"=w1736) -> ("Steps OUT"=w1735:string[])  [unwired: 9 in]
        n747 = Greater?(x=w1742, y=0.5) -> (0:w1743:bool)
        n748 = Index Array(array=w1735, index=1) -> (element=→"PCB":string)
        n749 = Bundle By Name(cluster=T19 {"DMM config cluster"={"DCV range"=0.0, "DCI range"=0.0, "Detector Rate"=0}, "mux2-1(DMM I) encode"=enum."DMM I (0.5)"} ("DMM all config"), "DMM config cluster.DCV range"=w1745, "DMM config cluster.DCI range"=w1742, "DMM config cluster.Detector Rate"=w1763) -> (w1767:T19)
        n750 = Select(t=enum16{"DMM I (0.5)", "DMM I (12)"}."DMM I (12)" ("mux2-1(DMM I) encode 2"), s=w1743, f=enum16{"DMM I (0.5)", "DMM I (12)"}."DMM I (0.5)" ("mux2-1(DMM I) encode 2")) -> (s? t:f=w1758:enum16{"DMM I (0.5)", "DMM I (12)"})
        n751 = To Variant(anything=w1767) -> (Variant=w1766:variant)
        n752 = To Variant(anything=w1758) -> (Variant=w1760:variant)
        n753 = call "App enquece.vi"("command data"=w1766, "command"="MEAS.Set DMM config", "queue in"=w1764) -> ("error out"=w1755:errorcluster, "Queue out"=w1759:refnum<queue>)  [unwired: 7 in]
        n754 = call "App enquece.vi"("error in (no error)"=w1755, "command data"=w1760, "command"="MEAS.Sel Input Current", "queue in"=w1759) -> ("error out"=w1741:errorcluster)  [unwired: 6 in, 1 out]
        n755 = Merge Errors(w1773, w1741) -> (w1762:errorcluster)
      }
      frame "INIT.Call DMM module" {
        n756 = disable-structure shown="LOGGING==TRUE" {
          disable-tunnel: w1786 -> [w1804 _]
          frame condition #0 (active) {
            n757 = Empty String/Path?(string/path=w1804) -> (empty?=w1807:bool)
            n758 = Select(t="Quece timeout", s=w1807, f=w1804) -> (s? t:f=w1803:string)
            n759 = call "string log (SubVI).vi"("Enum"=enum16{"Init", "Log", "Read"}."Log", "state Name"=w1803) -> ()  [unwired: 8 in, 2 out]
          }
          frame condition #1 {
          }
        }
        n760 = Unbundle By Name(w1797) -> ("HW config 2.DMM"=w1796:string)
        n761 = Type Cast(type=refnum<visa-resource-name> refnum ("VISA resource name 2"), x=w1796) -> (*(type *) &x=w1794:refnum<visa-resource-name>)
        n762 = call "Start Module.vi"("VISA resource name 2"=w1794) -> ("error out"=w1799:errorcluster, "Wait for Event Sync?"=w1793:bool, "DMM Module Broadcast Events"=w1792:T15)  [unwired: 7 in, 1 out]
        n763 = register-events(reference=w1800, w1792) -> (reference out=w1801:refnum<event-registration>)  [unwired: 5 in, 1 out]
        n764 = call "Synchronize Module Events.vi"("error in"=w1799, "Wait for Event Sync?"=w1793) -> ("error out"=w1798:errorcluster)  [unwired: 9 in]
        n765 = Merge Errors(w1787, w1798) -> (w1788:errorcluster)
      }
      frame "INIT.Call MUX module" {
        n766 = disable-structure shown="LOGGING==TRUE" {
          disable-tunnel: w1809 -> [w1827 _]
          frame condition #0 (active) {
            n767 = Empty String/Path?(string/path=w1827) -> (empty?=w1830:bool)
            n768 = Select(t="Quece timeout", s=w1830, f=w1827) -> (s? t:f=w1826:string)
            n769 = call "string log (SubVI).vi"("Enum"=enum16{"Init", "Log", "Read"}."Log", "state Name"=w1826) -> ()  [unwired: 8 in, 2 out]
          }
          frame condition #1 {
          }
        }
        n770 = Unbundle By Name(w1821) -> ("HW config 2.mux"=w1820:string)
        n771 = Type Cast(type=refnum<visa-resource-name> refnum ("VISA resource name"), x=w1820) -> (*(type *) &x=w1819:refnum<visa-resource-name>)
        n772 = call "Start Module.vi"("VISA resource name"=w1819) -> ("error out"=w1822:errorcluster, "Wait for Event Sync?"=w1816:bool, "Switches Module Broadcast Events"=w1817:T13)  [unwired: 7 in, 1 out]
        n773 = register-events(reference=w1823, w1817) -> (reference out=w1824:refnum<event-registration>)  [unwired: 5 in, 1 out]
        n774 = call "Synchronize Module Events.vi"("error in"=w1822, "Wait for Event Sync?"=w1816) -> ("error out"=w1815:errorcluster)  [unwired: 9 in]
        n775 = Merge Errors(w1810, w1815) -> (w1811:errorcluster)
      }
      frame "INIT.Call DEMUX module" {
        n776 = disable-structure shown="LOGGING==TRUE" {
          disable-tunnel: w1832 -> [w1850 _]
          frame condition #0 (active) {
            n777 = Empty String/Path?(string/path=w1850) -> (empty?=w1853:bool)
            n778 = Select(t="Quece timeout", s=w1853, f=w1850) -> (s? t:f=w1849:string)
            n779 = call "string log (SubVI).vi"("Enum"=enum16{"Init", "Log", "Read"}."Log", "state Name"=w1849) -> ()  [unwired: 8 in, 2 out]
          }
          frame condition #1 {
          }
        }
        n780 = Unbundle By Name(w1843) -> ("HW config 2.demux"=w1842:string)
        n781 = Type Cast(type=refnum<visa-resource-name> refnum ("COMport name"), x=w1842) -> (*(type *) &x=w1841:refnum<visa-resource-name>)
        n782 = call "Start Module.vi"("COMport name"=w1841) -> ("error out"=w1844:errorcluster, "Wait for Event Sync?"=w1845:bool, "MB 01 switches Module Broadcast Events"=w1839:T14)  [unwired: 7 in, 1 out]
        n783 = call "Synchronize Module Events.vi"("error in"=w1844, "Wait for Event Sync?"=w1845) -> ("error out"=w1838:errorcluster)  [unwired: 9 in]
        n784 = register-events(reference=w1846, w1839) -> (reference out=w1847:refnum<event-registration>)  [unwired: 5 in, 1 out]
        n785 = Merge Errors(w1833, w1838) -> (w1834:errorcluster)
      }
      frame "INIT.Call EMIC modules" {
        n786 = disable-structure shown="LOGGING==TRUE" {
          disable-tunnel: w1857 -> [w1874 _]
          frame condition #0 (active) {
            n787 = Empty String/Path?(string/path=w1874) -> (empty?=w1877:bool)
            n788 = Select(t="Quece timeout", s=w1877, f=w1874) -> (s? t:f=w1873:string)
            n789 = call "string log (SubVI).vi"("Enum"=enum16{"Init", "Log", "Read"}."Log", "state Name"=w1873) -> ()  [unwired: 8 in, 2 out]
          }
          frame condition #1 {
          }
        }
        n790 = Unbundle By Name(w1864) -> ("HW config 2.eMIC1"=w1871:string, "HW config 2.eMIC2"=w1870:string, "HW config 2.eMIC3"=w1869:string, "HW config 2.eMIC4"=w1868:string, "HW config 2.eMIC5"=w1867:string, "HW config 2.eMIC6"=w1866:string)
        n791 = Build Array(w1871, w1870, w1869, w1868, w1867, w1866) -> (w1855:string[])
        n792 = for {
          shift-right: [w1887] -> w1863
          shift-left: w1865 -> [w1885]
          tunnel: w1855 -> [w1886] mode=indexing
          tunnel: [w1879] -> w1861 mode=indexing
          n793 = Type Cast(type=refnum<visa-resource-name> refnum ("VISA resource name"), x=w1886) -> (*(type *) &x=w1883:refnum<visa-resource-name>)
          n794 = call "Start Module.vi"("VISA resource name"=w1883) -> ("error out"=w1880:errorcluster, "Wait for Event Sync?"=w1878:bool, "CE14_v2 Broadcast Events"=w1882:T12, "Module ID"=w1881:i32)  [unwired: 7 in]
          n795 = register-events(reference=w1885, w1882) -> (reference out=w1887:refnum<event-registration>)  [unwired: 5 in, 1 out]
          n796 = call "Synchronize Module Events.vi"("error in"=w1880, "Wait for Event Sync?"=w1878, "Module ID in"=w1881) -> ("error out"=w1879:errorcluster)  [unwired: 7 in, 1 out]
        }
        n797 = Merge Errors(w1858, w1861) -> (w1856:errorcluster)
      }
      frame "INIT.Open COM DMM" {
        n798 = disable-structure shown="LOGGING==TRUE" {
          disable-tunnel: w1891 -> [w1903 _]
          frame condition #0 (active) {
            n799 = Empty String/Path?(string/path=w1903) -> (empty?=w1906:bool)
            n800 = Select(t="Quece timeout", s=w1906, f=w1903) -> (s? t:f=w1902:string)
            n801 = call "string log (SubVI).vi"("Enum"=enum16{"Init", "Log", "Read"}."Log", "state Name"=w1902) -> ()  [unwired: 8 in, 2 out]
          }
          frame condition #1 {
          }
        }
        n802 = call "DMM connect and reset.vi"() -> ("error out"=w1895:errorcluster)  [unwired: 11 in]
        n803 = Merge Errors(w1892, w1895) -> (w1889:errorcluster)
        n804 = flat-sequence {
          tunnel: [w1901] -> w1890
          tunnel: w1889 -> [w1901]
          frame #0 {
            n805 = Wait (ms)(milliseconds to wait=u32 70) -> ()  [unwired: 1 out]
          }
        }
      }
      frame "INIT.Open COM MUX" {
        n806 = disable-structure shown="LOGGING==TRUE" {
          disable-tunnel: w1910 -> [w1922 _]
          frame condition #0 (active) {
            n807 = Empty String/Path?(string/path=w1922) -> (empty?=w1925:bool)
            n808 = Select(t="Quece timeout", s=w1925, f=w1922) -> (s? t:f=w1921:string)
            n809 = call "string log (SubVI).vi"("Enum"=enum16{"Init", "Log", "Read"}."Log", "state Name"=w1921) -> ()  [unwired: 8 in, 2 out]
          }
          frame condition #1 {
          }
        }
        n810 = call "inst.Open.vi"() -> ("error out"=w1916:errorcluster)  [unwired: 11 in]
        n811 = Merge Errors(w1911, w1916) -> (w1908:errorcluster)
        n812 = flat-sequence {
          tunnel: [w1920] -> w1909
          tunnel: w1908 -> [w1920]
          frame #0 {
            n813 = Wait (ms)(milliseconds to wait=u32 70) -> ()  [unwired: 1 out]
          }
        }
      }
      frame "INIT.Open COM DEMUX" {
        n814 = disable-structure shown="LOGGING==TRUE" {
          disable-tunnel: w1929 -> [w1941 _]
          frame condition #0 (active) {
            n815 = Empty String/Path?(string/path=w1941) -> (empty?=w1944:bool)
            n816 = Select(t="Quece timeout", s=w1944, f=w1941) -> (s? t:f=w1940:string)
            n817 = call "string log (SubVI).vi"("Enum"=enum16{"Init", "Log", "Read"}."Log", "state Name"=w1940) -> ()  [unwired: 8 in, 2 out]
          }
          frame condition #1 {
          }
        }
        n818 = call "MB01 Open.vi"() -> ("error out"=w1934:errorcluster)  [unwired: 11 in]
        n819 = Merge Errors(w1930, w1934) -> (w1927:errorcluster)
        n820 = flat-sequence {
          tunnel: [w1939] -> w1928
          tunnel: w1927 -> [w1939]
          frame #0 {
            n821 = Wait (ms)(milliseconds to wait=u32 70) -> ()  [unwired: 1 out]
          }
        }
      }
      frame "INIT.Open COM EMIC" {
        n822 = disable-structure shown="LOGGING==TRUE" {
          disable-tunnel: w1948 -> [w1961 _]
          frame condition #0 (active) {
            n823 = Empty String/Path?(string/path=w1961) -> (empty?=w1964:bool)
            n824 = Select(t="Quece timeout", s=w1964, f=w1961) -> (s? t:f=w1960:string)
            n825 = call "string log (SubVI).vi"("Enum"=enum16{"Init", "Log", "Read"}."Log", "state Name"=w1960) -> ()  [unwired: 8 in, 2 out]
          }
          frame condition #1 {
          }
        }
